vi "ArmBegin.vi"(8 "error in (no error)":errorcluster) -> (0 "error out":errorcluster)   [LabVIEW 2023]
doc: "Arm begin\nOpens ArmLift motor\nInputs:\nNone\nOutputs:\nnone"
uses:
  <vilib>/Rock Robotics/SystemInterfaces/DIO/FPGA_DIOChannel.ctl
  <vilib>/Rock Robotics/WPI/ThirdParty/REV Robotics/REVLib/Typedef/Spark MAX Sensor Type.ctl
  <vilib>/Rock Robotics/WPI/ThirdParty/REV Robotics/REVLib/Typedef/Spark MAX Limit Direction.ctl
  <vilib>/Rock Robotics/WPI/ThirdParty/REV Robotics/REVLib/Typedef/Spark MAX Limit Switch Polarity.ctl
  <vilib>/Rock Robotics/WPI/ThirdParty/REV Robotics/REVLib/Typedef/Spark MAX Idle Mode.ctl
  <vilib>/Rock Robotics/WPI/ThirdParty/REV Robotics/REVLib/Typedef/Spark MAX Motor Type.ctl
  <vilib>/Rock Robotics/WPI/Switch/WPI_SwitchOpenLimit.vi
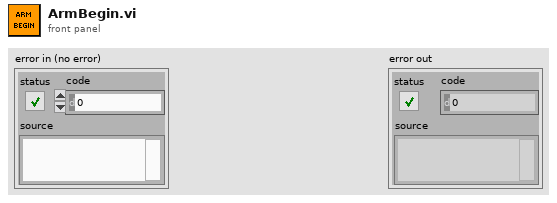
[diagram p1: front panel]
types:
  T1 = typedef "FPGA_DIOChannel.ctl" = enum8{"DIO 0", "DIO 1", "DIO 2", "DIO 3", "DIO 4", "DIO 5", "DIO 6", "DIO 7", "DIO 8", "DIO 9", "DIO MXP 0", "DIO MXP 1", "DIO MXP 2", "DIO MXP 3", "DIO MXP 4", "DIO MXP 5", "DIO MXP 6", "DIO MXP 7", "DIO MXP 8", "DIO MXP 9", "DIO MXP 10", "DIO MXP 11", "DIO MXP 12", "DIO MXP 13", "DIO MXP 14", "DIO MXP 15", "SPI Port CS1", "SPI Port CS2", "SPI Port CS3", "SPI Port MISO", "SPI Port MOSI", "Invalid"}
  T2 = typedef "Spark MAX Sensor Type.ctl" = enum16{"No Sensor", "Hall Sensor", "Encoder", "-Not Available-", "Analog", "Alternate Encoder", "Duty Cycle"}
  T3 = typedef "Spark MAX Limit Switch Polarity.ctl" = enum16{"Normally Open", "Normally Closed"}
  T4 = typedef "Spark MAX Limit Direction.ctl" = enum16{"Forward Limit", "Reverse Limit"}
  T5 = typedef "Spark MAX Idle Mode.ctl" = enum16{"Coast", "Brake"}
  T6 = typedef "Spark MAX Motor Type.ctl" = enum16{"Brushed", "Brushless"}
  T7 = typedef "WPI_MotorControlDeviceRef.ctl" = cluster{"DeviceStatus":errorcluster, "Type":T8, "PWM":cluster{"PWM Channel":T9, "DeadBand":T10}, "CAN":cluster{"Device Number":u8, "SetOutput VI Ref":variant, "GetOutput VI Ref":variant, "Enable VI Ref":variant, "Disable VI Ref":variant, "Data":variant}, "Invert":bool, "DIO PWM":cluster{"PWM \"Enable\" Channel":T9, "DIOChannel":T1, "PWM Rate":dbl}}
  T8 = typedef "WPI_MotorControlType.ctl" = enum16{"PWM", "CAN", "DIO PWM"}
  T9 = typedef "FPGA_DIOPWMChannel.ctl" = enum8{"PWM 0", "PWM 1", "PWM 2", "PWM 3", "PWM 4", "PWM 5", "PWM 6", "PWM 7", "PWM 8", "PWM 9", "PWM MXP 0", "PWM MXP 1", "PWM MXP 2", "PWM MXP 3", "PWM MXP 4", "PWM MXP 5", "PWM MXP 6", "PWM MXP 7", "PWM MXP 8", "PWM MXP 9", "Invalid"}
  T10 = typedef "WPI_PWMDeadband.ctl" = cluster{"Name":string, "maxPositivePwm":i32, "minPositivePwm":i32, "centerPwm":i32, "maxNegativePwm":i32, "minNegativePwm":i32, "angularRange":u16}
  T11 = typedef "WPI_SwitchDevRef.ctl" = cluster{"DevStatus":errorcluster, "DIO Channel":T1, "CntIndex":T12, "Normally Closed":bool}
  T12 = typedef "FPGA_CounterCtrSystemIndex.ctl" = enum8{"Ctr 0", "Ctr 1", "Ctr 2", "Ctr 3", "Ctr 4", "Ctr 5", "Ctr 6", "Ctr 7", "Invalid"}
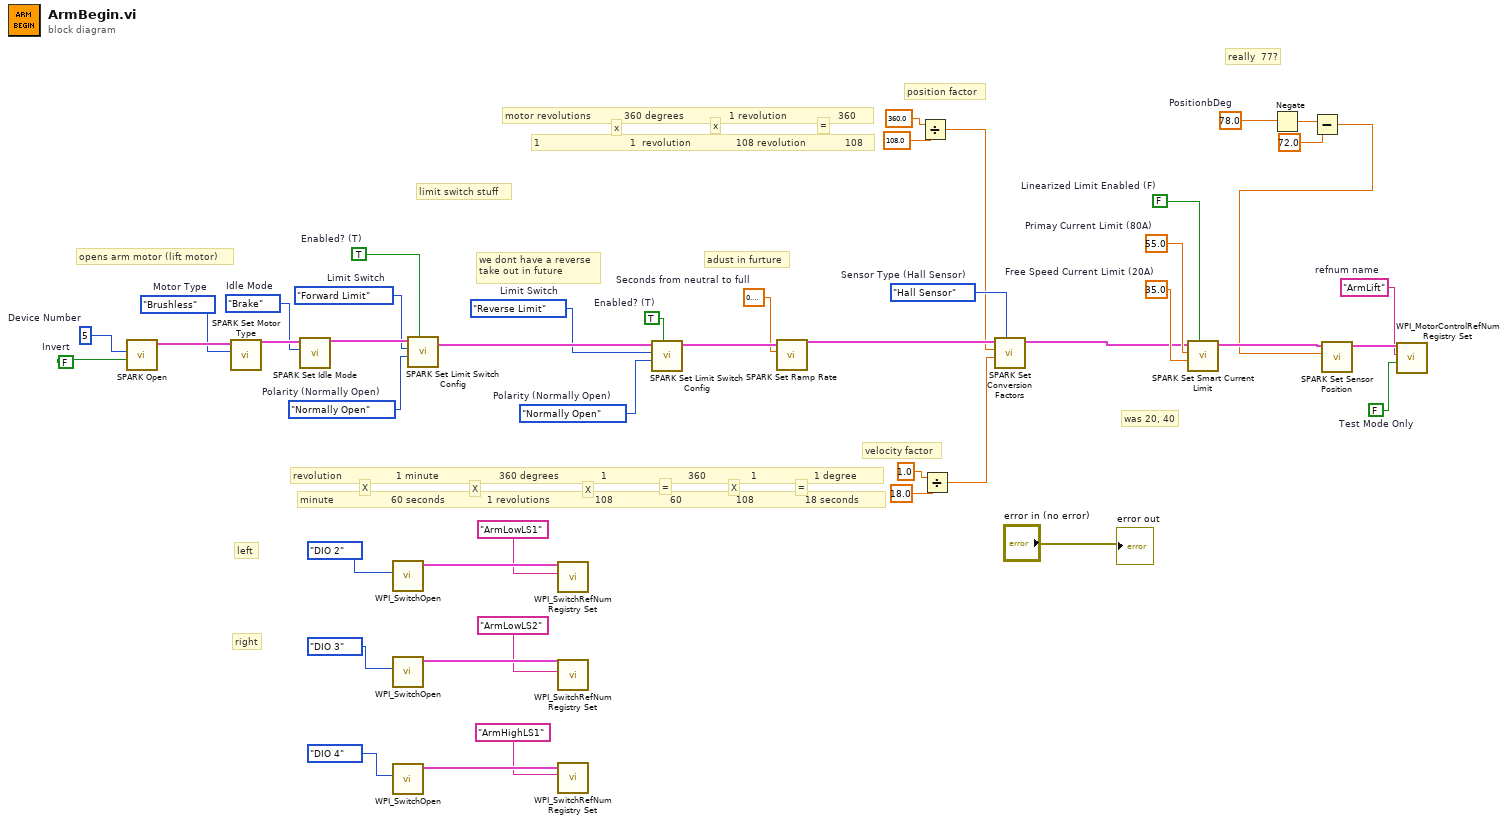
[diagram p0: block diagram]
diagram:
  w17 = FALSE  # Test Mode Only
  w22 = FALSE  # Linearized Limit Enabled (F)
  w24 = Spark_MAX_Sensor_Type."Hall Sensor"  # Sensor Type (Hall Sensor)
  w26 = sgl 0.2  # Seconds from neutral to full
  w28 = Spark_MAX_Limit_Switch_Polarity."Normally Open"  # Polarity (Normally Open)
  w29 = TRUE  # Enabled? (T)
  w30 = Spark_MAX_Limit_Direction."Reverse Limit"  # Limit Switch
  w32 = Spark_MAX_Limit_Switch_Polarity."Normally Open"  # Polarity (Normally Open)
  w33 = TRUE  # Enabled? (T)
  w34 = Spark_MAX_Limit_Direction."Forward Limit"  # Limit Switch
  w13 = 78.0  # PositionbDeg
  w36 = "ArmLift"  # refnum name
  w39 = 35.0  # Free Speed Current Limit (20A)
  w40 = 55.0  # Primay Current Limit (80A)
  w41 = Spark_MAX_Idle_Mode."Brake"  # Idle Mode
  w43 = Spark_MAX_Motor_Type."Brushless"  # Motor Type
  w45 = FALSE  # Invert
  w46 = u8 5  # Device Number
  # "right"
  # "left"
  # "was 20, 40"
  # "we dont have a reverse\ntake out in future"
  # "adust in furture"
  # "velocity factor"
  # "position factor"
  # "limit switch stuff"
  # "X"
  # "X"
  # "X"
  # "X"
  # "="
  # "="
  # "minute                   60 seconds              1 revolutions               108                   60                  108                 18 seconds"
  # "revolution                  1 minute                    360 degrees              1                           360               1                   1 degree"
  # "1                              1  revolution               108 revolution             108"
  # "="
  # "x"
  # "x"
  # "motor revolutions           360 degrees               1 revolution                 360"
  # "really  77?"
  # "opens arm motor (lift motor)"
  n1 = call <vilib>:"SPARK Open.vi"("Invert"=w45, "Device Number"=w46) -> ("MotorControlDeviceRef"=w44:T7)  [unwired: 8 in, 1 out]
  n2 = call <vilib>:"SPARK Set Motor Type.vi"("Motor Type"=w43, "MotorControlDevRef"=w44) -> ("MotorControlDeviceRef"=w42:T7)  [unwired: 8 in, 1 out]
  n3 = call <vilib>:"SPARK Set Idle Mode.vi"("Idle Mode"=w41, "MotorControlDeviceRef in"=w42) -> ("MotorControlDeviceRef out"=w35:T7)  [unwired: 8 in, 1 out]
  n4 = call-poly <vilib>:"WPI_SwitchOpen.vi"("DIO Channel"=FPGA_DIOChannel."DIO 2") -> ("SwitchDevRef"=w9:T11)  [unwired: 9 in, 1 out]
  n5 = call-poly <vilib>:"WPI_SwitchOpen.vi"("DIO Channel"=FPGA_DIOChannel."DIO 3") -> ("SwitchDevRef"=w3:T11)  [unwired: 9 in, 1 out]
  n6 = call-poly <vilib>:"WPI_SwitchOpen.vi"("DIO Channel"=FPGA_DIOChannel."DIO 4") -> ("SwitchDevRef"=w6:T11)  [unwired: 9 in, 1 out]
  n7 = call <vilib>:"SPARK Set Limit Switch Config.vi"("Enabled? (T)"=w33, "Polarity (Normally Open)"=w32, "Limit Switch"=w34, "MotorControlDeviceRef in"=w35) -> ("MotorControlDeviceRef out"=w31:T7)  [unwired: 6 in, 1 out]
  n8 = call <vilib>:"WPI_SwitchRefNum Registry Set.vi"("refnum name"="ArmLowLS1", "SwitchDevRef"=w9) -> ()  [unwired: 8 in, 2 out]
  n9 = call <vilib>:"WPI_SwitchRefNum Registry Set.vi"("refnum name"="ArmLowLS2", "SwitchDevRef"=w3) -> ()  [unwired: 8 in, 2 out]
  n10 = call <vilib>:"WPI_SwitchRefNum Registry Set.vi"("refnum name"="ArmHighLS1", "SwitchDevRef"=w6) -> ()  [unwired: 8 in, 2 out]
  n11 = call <vilib>:"SPARK Set Limit Switch Config.vi"("Enabled? (T)"=w29, "Polarity (Normally Open)"=w28, "Limit Switch"=w30, "MotorControlDeviceRef in"=w31) -> ("MotorControlDeviceRef out"=w27:T7)  [unwired: 6 in, 1 out]
  n12 = call <vilib>:"SPARK Set Ramp Rate.vi"("Seconds from neutral to full (0)"=w26, "MotorControlDeviceRef in"=w27) -> ("MotorControlDeviceRef"=w25:T7)  [unwired: 8 in, 1 out]
  n13 = Divide(x=360.0 ("Velocity Factor (1)"), y=108.0) -> (x/y=w15:dbl)
  n14 = Divide(x=1.0 ("Velocity Factor (1)"), y=18.0) -> (x/y=w14:dbl)
  n15 = call <vilib>:"SPARK Set Conversion Factors.vi"("Sensor Type (Hall Sensor)"=w24, "Velocity Factor (1)"=w14, "Position Factor (1)"=w15, "MotorControlDeviceRef in"=w25) -> ("MotorControlDeviceRef out"=w23:T7)  [unwired: 6 in, 1 out]
  n16 = call <vilib>:"SPARK Set Smart Current Limit.vi"("Linearized Limit Enabled (F)"=w22, "Free Speed Current Limit (20A)"=w39, "Primay Current Limit (80A)"=w40, "MotorControlDeviceRef in"=w23) -> ("MotorControlDeviceRef out"=w38:T7)  [unwired: 6 in, 1 out]
  n17 = Negate(x=w13) -> (-x=w12:dbl)
  n18 = Subtract(x=w12, y=72.0) -> (x-y=w10:dbl)
  n19 = call <vilib>:"SPARK Set Sensor Position.vi"("Position"=w10, "MotorControlDeviceRef"=w38) -> ("MotorControlDeviceRef"=w37:T7)  [unwired: 8 in, 1 out]
  n20 = call <vilib>:"WPI_MotorControlRefNum Registry Set.vi"("Test Mode Only"=w17, "refnum name"=w36, "MotorControlDevRef"=w37) -> ()  [unwired: 7 in, 2 out]
  "error out" <- "error in (no error)"
